vi "configuration.get.vi"(11 "configuration-data in":refnum<class "configuration-data.lvclass">) -> (2 "configuration":T1)   [LabVIEW 2020, in "configuration-data.lvclass"]
uses:
  configuration-data.lvclass
  configuration--map.ctl
  value--cluster.ctl
  datatype--enum.ctl
  configuration-data.lvclass/configuration-data.ctl
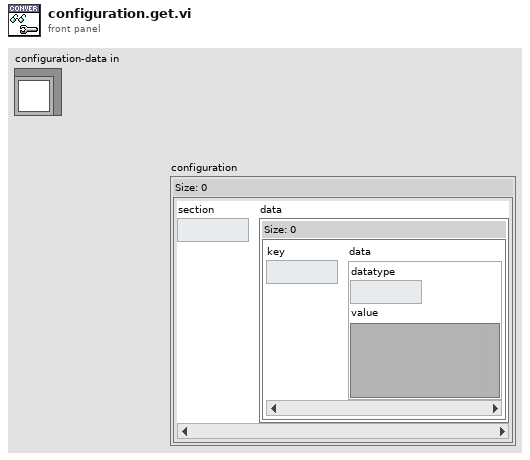
[diagram p1: front panel]
types:
  T1 = typedef "configuration-data.lvclass/configuration--map.ctl" = map{string, map{string, T2}}
  T2 = typedef "configuration-data.lvclass/value--cluster.ctl" = cluster{"datatype":T3, "value":variant}
  T3 = typedef "configuration-data.lvclass/datatype--enum.ctl" = enum16{"Boolean", "Double", "Integer", "String"}
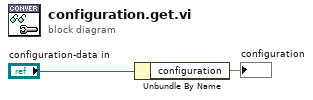
[diagram p0: block diagram]
diagram:
  n1 = Unbundle By Name("configuration-data in") -> ("configuration"=→"configuration":T1)
